vi "UI Subpanel.vi"() -> ()   [LabVIEW 2021, in "CIF Core UI.lvlib"]
uses:
  CIF Core UI.lvlib
  CIFUI/Typedef/Class Data for SubPanel.ctl
  <vilib>/gRPC/LabVIEW gRPC Library/Shared/grpcId.ctl
  CIFUI/Typedef/Core UI References.ctl
  CIFUI/Typedef/Channel Connection.ctl
  CIFUI/Typedef/New Plugin.ctl
  CIFUI/Typedef/Run Listen Button.ctl
  CIFUI/Typedef/CIF_Manager_UI_Tab.ctl
  CIFUI/Typedef/SubPanel Events.ctl
  CIFUI/Typedef/New Connection Event Data.ctl
  CIFUI/Typedef/New Connection Plugin Event Data.ctl
  Common/Typedef/Common Plugin Configuration.ctl
  Common/Typedef/External Clock Config.ctl
  CIFUI/CIF_UI.lvclass
  CIFUI/CIF_UI.lvclass/CIF_UI.ctl
  CIFUI/Utilities/Get Human Readable Error.vi
  <vilib>/CIF Foundation/CIF Utilities/Errors/Append Error Location.vi
  <vilib>/CIF Foundation/CIF Utilities/Errors/Human Readable Error Message.vi
  Grpc/CIFCoreWrapper/CIFCoreWrapper.lvlib
  <vilib>/addons/_JKI.lib/Serialization/JSON/JKI JSON Serialization.lvlib
  Common/CIFCoreCommon.lvlib
  <vilib>/gRPC/LabVIEW gRPC Library/grpc-lvsupport-release.lvlib
panel:
  in  "Configuration":cluster{"Common":T1}={"Common"={"Period (s)"=0.001, "Offset (us)"=0, "Priority"=100, "Processor"=-2, "External Clock"={"ClockID"=0, "Clock Name"="", "Publish Clock"=FALSE, "Convert Data Timestamps"=FALSE, "Plugin Timing Source"=FALSE}}} {"Common"."Period (s)" format="%#_13g"}
  in  "Class Data for SubPanel":T3
  in  "Update Config":bool
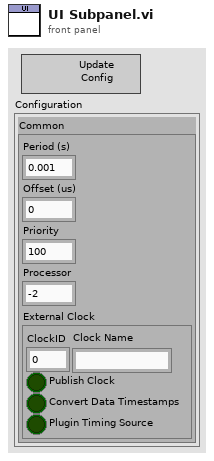
[diagram p1: front panel]
types:
  T1 = typedef "CIFCoreCommon.lvlib/Common Plugin Configuration.ctl" = cluster{"Period (s)":dbl, "Offset (us)":i32, "Priority":i32, "Processor":i32, "External Clock":T2}
  T2 = typedef "CIFCoreCommon.lvlib/External Clock Config.ctl" = cluster{"ClockID":u8, "Clock Name":string, "Publish Clock":bool, "Convert Data Timestamps":bool, "Plugin Timing Source":bool}
  T3 = typedef "CIF_UI.lvclass/Class Data for SubPanel.ctl" = cluster{"IP Address":string, "Manager gRPC ID":T4, "Server Certificate File (.crt)":path, "Connected":bool, "Manager Connection":bool, "Core UI References":T5, "Subpanel Events":T6}
  T4 = typedef "grpc-lvsupport-release.lvlib/grpcId.ctl" = u64
  T5 = typedef "CIF_UI.lvclass/Core UI References.ctl" = cluster{"Discovered Plugins":refnum<vi>, "Discovered Plugins Valid":bool, "Loaded Plugins":refnum<vi>, "Loaded Plugins Valid":bool, "Publisher Channels":refnum<vi>, "Publisher Channels Valid":bool, "Subscriber Channels":refnum<vi>, "Subscriber Channels Valid":bool, "Plugin Status":refnum<vi>, "Plugin Status Valid":bool, "Channel Connection":refnum<vi>, "Channel Connection Valid":bool, "New Plugin Load":refnum<vi>, "New Plugin Load Valid":bool, "Errors":refnum<vi>, "Errors Valid":bool, "Plugin to Abort":refnum<vi>, "Plugin to Abort Valid":bool, "Connection":refnum<vi>, "Connection Valid":bool, "Exit":refnum<vi>, "Exit Valid":bool, "Run Listen":refnum<vi>, "Run Listen Valid":bool, "CIF Manager Tab":refnum<vi>, "Manger Tab Valid":bool, "Clear Local Error":refnum<vi>, "Clear Local Error Valid":bool, "Local Error":refnum<vi>, "Local Error Valid":bool, "System Errors":refnum<vi>, "System Errors Valid":bool, "Plugin Selection":refnum<vi>, "Plugin Selection Valid":bool}
  T6 = typedef "CIF_UI.lvclass/SubPanel Events.ctl" = cluster{"Clear Local Error":refnum<user-event>, "Shutdown":refnum<user-event>, "gRPC Connection":refnum<user-event>, "Plugin Connection":refnum<user-event>}
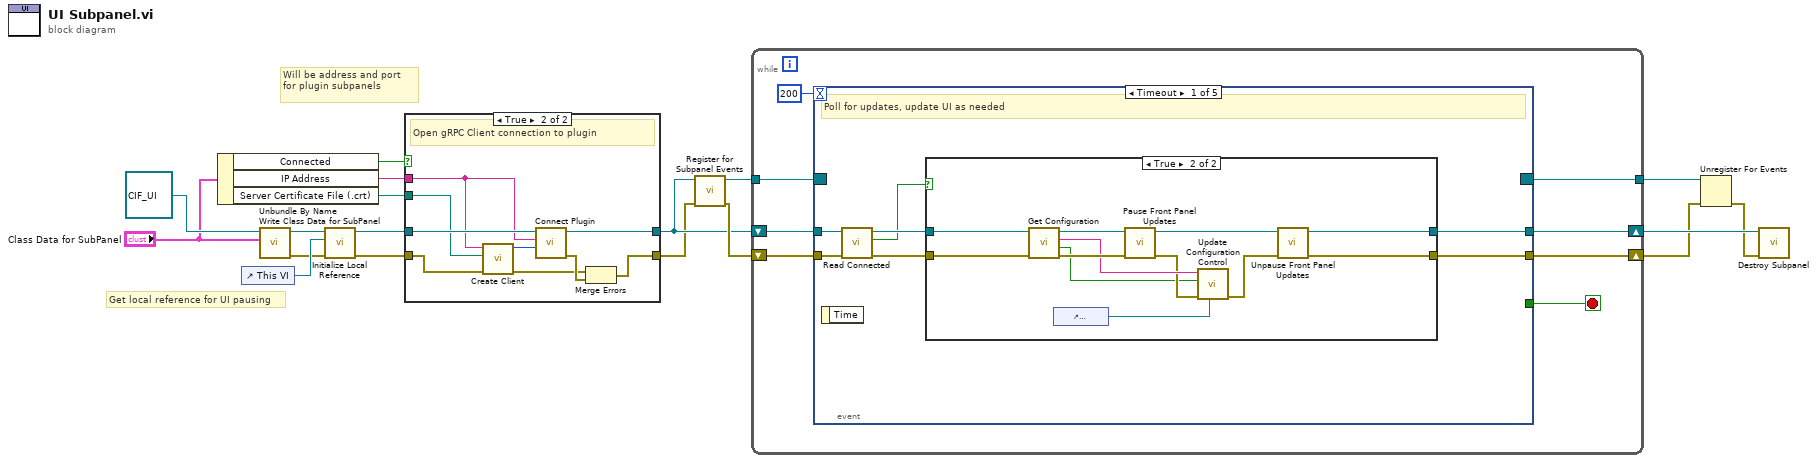
[diagram p0: block diagram]
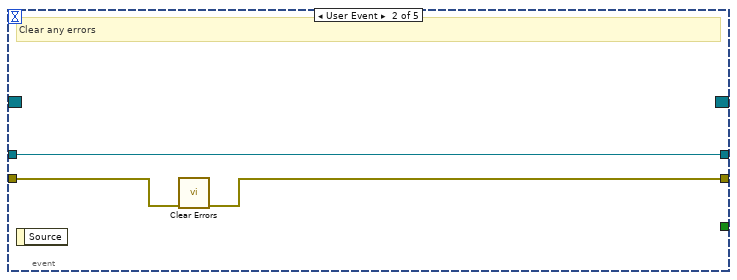
[diagram p4: hidden frame]
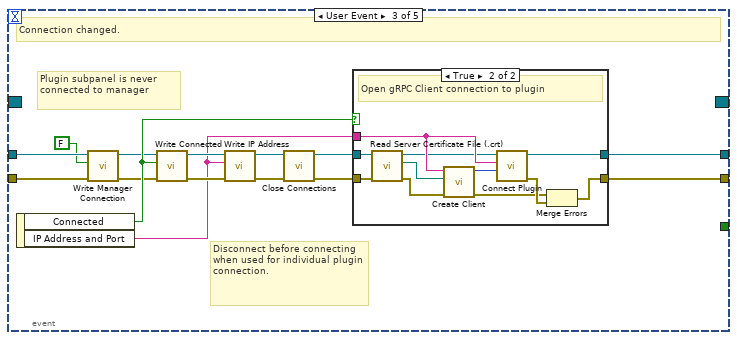
[diagram p5: hidden frame]
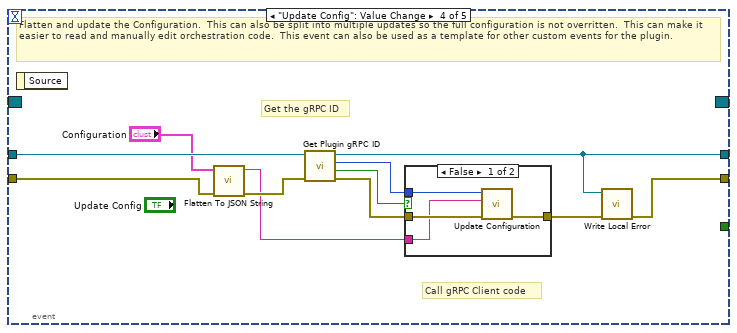
[diagram p7: hidden frame]
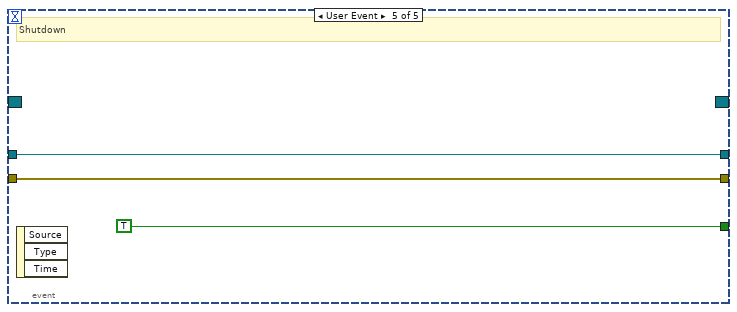
[diagram p9: hidden frame]
diagram:
  # "Will be address and port for plugin subpanels"
  # "Get local reference for UI pausing"
  n1 = Unbundle By Name("Class Data for SubPanel") -> ("Connected"=w3:bool, "IP Address"=w2:string, "Server Certificate File (.crt)"=w1:path)
  n2 = control-ref of="This VI"() -> (w18:refnum<vi>)
  n3 = call "Write Class Data for SubPanel.vi"("Class Data for SubPanel"="Class Data for SubPanel", "CIF_UI in"=refnum<class "CIF_UI.lvclass"> refnum) -> ("error out"=w9:errorcluster, "CIF_UI out"=w11:refnum<class "CIF_UI.lvclass">)  [unwired: 8 in]
  n4 = call "Initialize Local Reference.vi"("error in (no error)"=w9, "This VI"=w18, "CIF_UI in"=w11) -> ("error out"=w7:errorcluster, "CIF_UI out"=w8:refnum<class "CIF_UI.lvclass">)  [unwired: 7 in]
  n5 = case shown="True" w3 {
    tunnel: [w19 w29] -> w5
    tunnel: [w20 w27] -> w6
    tunnel: w8 -> [w20 w26]
    tunnel: w7 -> [w19 w25]
    tunnel: w2 -> [_ w22]
    tunnel: w1 -> [_ w21]
    frame False {
    }
    frame True {
      # "Open gRPC Client connection to plugin"
      n6 = call "Create Client.vi"("error in"=w25, "Server Certificate File (.crt)"=w21, "address"=w22) -> ("error out"=w24:errorcluster, "gRPC ID Out"=w23:T4)  [unwired: 7 in]
      n7 = call "Connect Plugin.vi"("gRPC ID"=w23, "Address"=w22, "CIF_UI in"=w26) -> ("error out"=w28:errorcluster, "CIF_UI out"=w27:refnum<class "CIF_UI.lvclass">)  [unwired: 7 in]
      n8 = Merge Errors(w24, w28) -> (w29:errorcluster)
    }
  }
  n9 = call "Register for Subpanel Events.vi"("error in (no error)"=w5, "CIF_UI in"=w6) -> ("error out"=w16:errorcluster, "Event Registration Refnum"=w17:refnum<event-registration>)  [unwired: 8 in]
  n10 = while {
    tunnel: w17 -> [w36]
    shift-right: [w31] -> w15
    shift-left: w6 -> [w34]
    shift-right: [w32] -> w13
    shift-left: w16 -> [w33]
    tunnel: [w30] -> w14
    stop <- w35 stop-if-true
    n11 = event shown="[0] Timeout" {
      selector: w36 -> [_ _ _ _ _]
      dyn-events: [_ _ _ _ _] -> w30
      timeout: 200 -> [_ _ _ _ _]
      tunnel: [_ _ _ _ TRUE] -> w35
      tunnel: w34 -> [w40 w59 w66 w96 w107]
      tunnel: w33 -> [w41 w61 w65 w100 w106]
      tunnel: [w38 w60 w67 w90 w106] -> w32
      tunnel: [w39 w59 w68 w91 w107] -> w31
      event Timeout {
        # "Poll for updates, update UI as needed"
        n12 = event-data() -> ()  [unwired: 1 in, 1 out]
        n13 = call "Read Connected.vi"("error in (no error)"=w41, "CIF_UI in"=w40) -> ("error out"=w43:errorcluster, "Connected"=w42:bool, "CIF_UI out"=w44:refnum<class "CIF_UI.lvclass">)  [unwired: 7 in]
        n14 = case shown="True" w42 {
          tunnel: w43 -> [w45 w55]
          tunnel: [w45 w58] -> w38
          tunnel: w44 -> [w46 w56]
          tunnel: [w46 w57] -> w39
          frame False {
          }
          frame True {
            n15 = call "Get Configuration.vi"("error in (no error)"=w55, "CIF_Plugin_UI in"=w56) -> ("error out"=w53:errorcluster, "Not Found"=w48:bool, "JSON Configuration"=w51:string, "CIF_Plugin_UI out"=w54:refnum<class "CIF_UI.lvclass">)  [unwired: 6 in]
            n16 = control-ref of="Configuration"() -> (w49:refnum<vi>)
            n17 = call "Pause Front Panel Updates.vi"("error in (no error)"=w53, "CIF_UI in"=w54) -> ("error out"=w50:errorcluster, "CIF_UI out"=w52:refnum<class "CIF_UI.lvclass">)  [unwired: 8 in]
            n18 = call "Update Configuration Control.vi"("Configuration reference"=w49, "error in (no error)"=w50, "Not Valid"=w48, "JSON Configuration"=w51) -> ("error out"=w47:errorcluster)  [unwired: 7 in]
            n19 = call "Unpause Front Panel Updates.vi"("error in (no error)"=w47, "CIF_UI in"=w52) -> ("error out"=w58:errorcluster, "CIF_UI out"=w57:refnum<class "CIF_UI.lvclass">)  [unwired: 8 in]
          }
        }
      }
      event User Event {
        # "Clear any errors"
        n20 = event-data() -> ()  [unwired: 1 in, 1 out]
        n21 = call <vilib>:"Clear Errors.vi"("error in (no error)"=w61) -> ("error out"=w60:errorcluster)  [unwired: 5 in, 1 out]
      }
      event User Event {
        # "Plugin subpanel is never connected to manager"
        # "Disconnect before connecting when used for individual plugin connection."
        # "Connection changed."
        n22 = event-data() -> ("Connected"=w69:bool, "IP Address and Port"=w70:string)  [unwired: 1 in]
        n23 = call "Write Manager Connection.vi"("error in (no error)"=w65, "Manager Connection"=FALSE, "CIF_UI in"=w66) -> ("error out"=w63:errorcluster, "CIF_UI out"=w64:refnum<class "CIF_UI.lvclass">)  [unwired: 7 in]
        n24 = call "Write Connected.vi"("error in (no error)"=w63, "Connected"=w69, "CIF_UI in"=w64) -> ("error out"=w75:errorcluster, "CIF_UI out"=w76:refnum<class "CIF_UI.lvclass">)  [unwired: 7 in]
        n25 = call "Write IP Address.vi"("error in (no error)"=w75, "IP Address"=w70, "CIF_UI in"=w76) -> ("error out"=w73:errorcluster, "CIF_UI out"=w74:refnum<class "CIF_UI.lvclass">)  [unwired: 7 in]
        n26 = call "Close Connections.vi"("error in (no error)"=w73, "CIF_UI in"=w74) -> ("error out"=w71:errorcluster, "CIF_UI out"=w72:refnum<class "CIF_UI.lvclass">)  [unwired: 8 in]
        n27 = case shown="True" w69 {
          tunnel: [w77 w89] -> w67
          tunnel: [w78 w87] -> w68
          tunnel: w72 -> [w78 w83]
          tunnel: w71 -> [w77 w82]
          tunnel: w70 -> [_ w84]
          frame False {
          }
          frame True {
            # "Open gRPC Client connection to plugin"
            n28 = call "Read Server Certificate File (.crt).vi"("error in (no error)"=w82, "CIF_UI in"=w83) -> ("error out"=w80:errorcluster, "Server Certificate File (.crt)"=w79:path, "CIF_UI out"=w81:refnum<class "CIF_UI.lvclass">)  [unwired: 7 in]
            n29 = call "Create Client.vi"("error in"=w80, "Server Certificate File (.crt)"=w79, "address"=w84) -> ("error out"=w86:errorcluster, "gRPC ID Out"=w85:T4)  [unwired: 7 in]
            n30 = call "Connect Plugin.vi"("gRPC ID"=w85, "Address"=w84, "CIF_UI in"=w81) -> ("error out"=w88:errorcluster, "CIF_UI out"=w87:refnum<class "CIF_UI.lvclass">)  [unwired: 7 in]
            n31 = Merge Errors(w86, w88) -> (w89:errorcluster)
          }
        }
      }
      event "Update Config": Value Change {
        # "Call gRPC Client code"
        # "Get the gRPC ID"
        # "Flatten and update the Configuration.  This can also be split into multiple updates so the full configuration is not overritten.  This can make it easier to read and manually edit orchestration code.  This event can also be used as a template for other custom events for the plugin."
        n32 = event-data() -> ()  [unwired: 1 in, 1 out]
        n33 = call <vilib>:"Flatten To JSON String.vi"("error in (no error)"=w100, "Variant"="Configuration") -> ("error out"=w95:errorcluster, "JSON String"=w94:string)  [unwired: 8 in]
        n34 = call "Get Plugin gRPC ID.vi"("error in (no error)"=w95, "CIF_UI in"=w96) -> ("error out"=w97:errorcluster, "Not Found"=w98:bool, "gRPC ID"=w99:T4, "CIF_UI out"=w91:refnum<class "CIF_UI.lvclass">)  [unwired: 5 in, 1 out]
        n35 = case shown="False" w98 {
          tunnel: w99 -> [w104 _]
          tunnel: w97 -> [w103 w105]
          tunnel: [w102 w105] -> w92
          tunnel: w94 -> [w101 _]
          frame False {
            n36 = call "Update Configuration.vi"("error in"=w103, "JSON Configuration"=w101, "gRPC ID"=w104) -> ("error out"=w102:errorcluster)  [unwired: 7 in, 1 out]
          }
          frame True {
          }
        }
        n37 = call "Write Local Error.vi"("error in (no error)"=w92, "CIF_UI in"=w91) -> ("error out"=w90:errorcluster)  [unwired: 9 in]
      }
      event User Event {
        # "Shutdown"
        n38 = event-data() -> ()  [unwired: 1 in, 3 out]
      }
    }
  }
  n39 = Unregister For Events(event registration refnum=w14, error in=w13) -> (error out=w12:errorcluster)
  n40 = call "Destroy Subpanel.vi"("error in (no error)"=w12, "CIF_UI in"=w15) -> ()  [unwired: 8 in, 2 out]
